vi "Edit_Manual_ADAM_Chs.vi"(3 "Mode":enum16{"Load from File", "Save to File"}(ring)=enum."Save to File", 4 "Documentation level In":T1, 5 "Channel Names In":string[](array[string])) -> (1 "Documentation level Out":T1, 2 "Channel Names Out":string[](array[string]))   [LabVIEW 2010]
uses:
  Gen Trav/Documentation.ctl
  Globals/Constants_global.vi
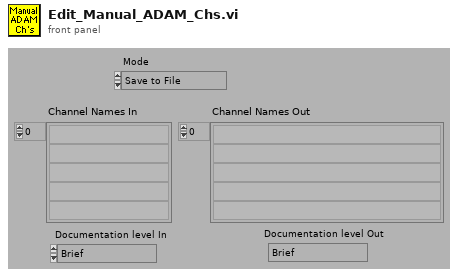
[diagram p1: front panel]
types:
  T1 = typedef "Documentation.ctl" = enum16{"Brief", "Full", "All Active channels"}
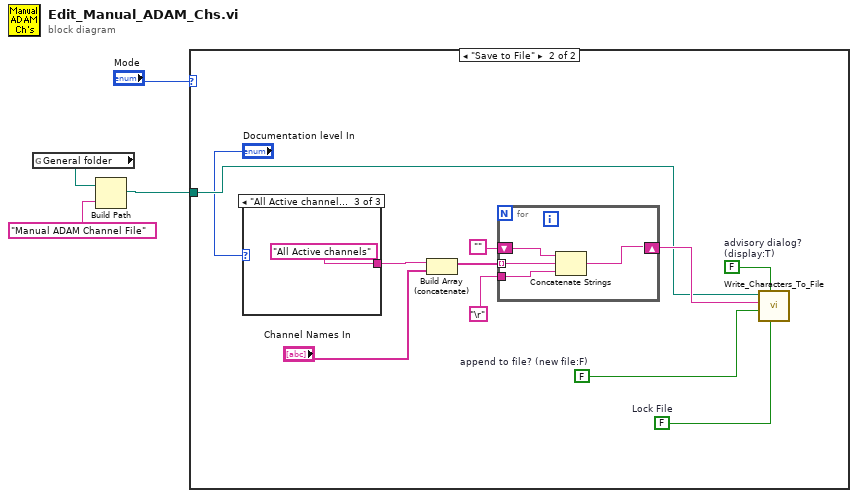
[diagram p0: block diagram]
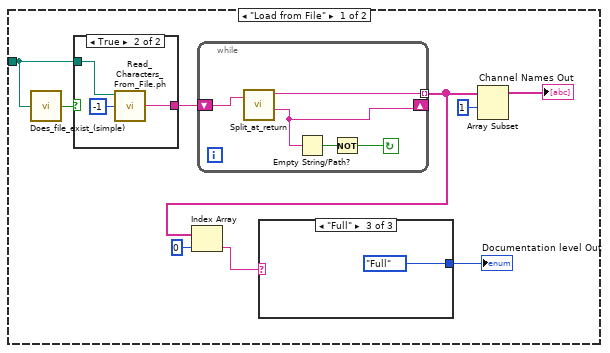
[diagram p2: hidden frame]
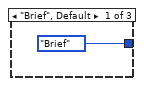
[diagram p3: hidden frame]
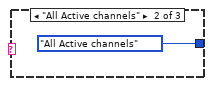
[diagram p4: hidden frame]
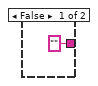
[diagram p5: hidden frame]
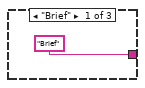
[diagram p6: hidden frame]
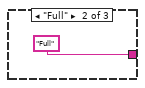
[diagram p7: hidden frame]
diagram:
  n1 = global read "Constants_global.vi" "General folder"() -> (w3:path)
  n2 = Build Path(base path=w3, name or relative path="Manual ADAM Channel File" ("Substring")) -> (appended path=w1:path)
  n3 = case shown="\"Save to File\"" "Mode" {
    tunnel: w1 -> [w13 w33]
    frame "Load from File" {
      n4 = call "Does_file_exist_(simple).vi"("Pathname"=w13) -> ("exists?"=w12:bool)
      n5 = case shown="True" w12 {
        tunnel: ["" ("character string") w24] -> w11
        tunnel: w13 -> [_ w23]
        frame False {
        }
        frame True {
          n6 = call "Read_Characters_From_File.ph.vi"("file path (dialog if empty)"=w23, "number of characters (all:-1)"=-1) -> ("character string"=w24:string)  [unwired: 4 in, 3 out]
        }
      }
      n7 = while {
        shift-left: w11 -> [w15]
        shift-right: [w14] -> _
        tunnel: [w18] -> w8 mode=indexing
        stop <- w16 continue-if-true
        n8 = call "Split_at_return.vi"("String"=w15) -> ("before substring"=w18:string, "after substring"=w14:string)  [unwired: 1 in, 2 out]
        n9 = Empty String/Path?(string/path=w14) -> (empty?=w17:bool)
        n10 = Not(x=w17) -> (.not. x?=w16:bool)
      }
      n11 = Index Array(array=w8, index=0 ("Index")) -> (element=w5:string)
      n12 = case shown="\"Full\"" w5 {
        tunnel: [Documentation."Brief" ("Documentation level Out") Documentation."All Active channels" ("Documentation level Out") Documentation."Full" ("Documentation level Out")] -> w6
        frame "Brief", Default {
        }
        frame "All Active channels" {
        }
        frame "Full" {
        }
      }
      "Documentation level Out" <- w6
      n13 = Array Subset(array=w8, index=1 ("Array Index")) -> (→"Channel Names Out":string[])  [unwired: 1 in]
    }
    frame "Save to File" {
      w26 = FALSE  # Lock File
      w31 = FALSE  # append to file? (new file:F)
      w32 = FALSE  # advisory dialog? (display:T)
      n14 = case shown="\"All Active channels\"" "Documentation level In" {
        tunnel: ["Brief" "Full" "All Active channels"] -> w28
        frame "Brief" {
        }
        frame "Full" {
        }
        frame "All Active channels" {
        }
      }
      n15 = Build Array (concatenate)(w28, "Channel Names In") -> (w27:string[])
      n16 = for {
        tunnel: w27 -> [w43] mode=indexing
        tunnel: "\r" -> [w42]
        shift-right: [w40] -> w34
        shift-left: "" -> [w41]
        n17 = Concatenate Strings(w41, w43, w42) -> (w40:string)
      }
      n18 = call "Write_Characters_To_File.vi"("file path (dialog if empty)"=w33, "advisory dialog? (display:T)"=w32, "character string"=w34, "append to file? (new file:F)"=w31, "Lock File"=w26) -> ()  [unwired: 3 in, 1 out]
    }
  }
